vi "Scale Cartesian Coordinates 2D.vi"(3 "Max Radius":dbl, 5 "Source Coordinates (cm, cm)":cluster{"x":dbl, "y":dbl}={"x"=59.5, "y"=52.5}) -> (1 "output cluster":cluster{"x":dbl, "y":dbl})   [LabVIEW 2013]
panel:
  out "output variable":dbl
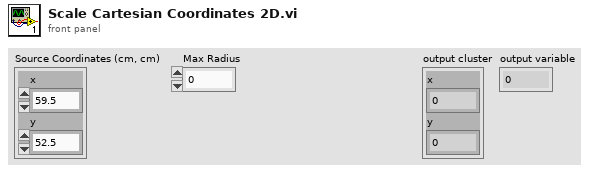
[diagram p1: front panel]
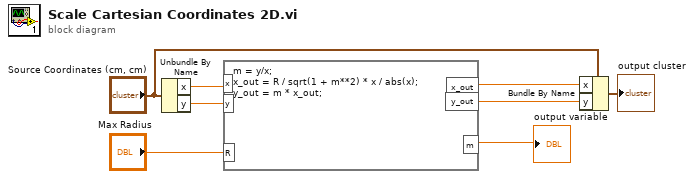
[diagram p0: block diagram]
diagram:
  n1 = Unbundle By Name("Source Coordinates (cm, cm)") -> ("x"=w8:dbl, "y"=w7:dbl)
  n2 = formula code="m = y/x;\nx_out = R / sqrt(1 + m**2) * x / abs(x);\ny_out = m * x_out;"("R"="Max Radius", "x"=w8, "y"=w7) -> ("x_out"=w3:dbl, "m"=→"output variable":dbl, "y_out"=w1:dbl)
  n3 = Bundle By Name(cluster="Source Coordinates (cm, cm)", "x"=w3, "y"=w1) -> (→"output cluster":cluster{"x":dbl, "y":dbl})
